vi "test_Error Code Channel Waveform Outgoing.vi"(8 "error in (no error)":errorcluster, 11 "TestCase in":refnum<class "FPGA Addon DMA Waveform Status Channel System Tests.lvclass">) -> (0 "error out":errorcluster, 3 "TestCase out":refnum<class "FPGA Addon DMA Waveform Status Channel System Tests.lvclass">)   [LabVIEW 2018, in "FPGA Addon DMA Waveform Status Channel System Tests.lvclass"]
uses:
  FPGA Addon DMA Waveform Status Channel System Tests.lvclass
  <vilib>/addons/_JKI Toolkits/VI Tester/TestCase.llb/TestCase.lvclass
  C:/Program Files (x86)/National Instruments/LabVIEW 2018/vi.lib/addons/_JKI Toolkits/VI Tester/TestCase.llb/TestCase.lvclass
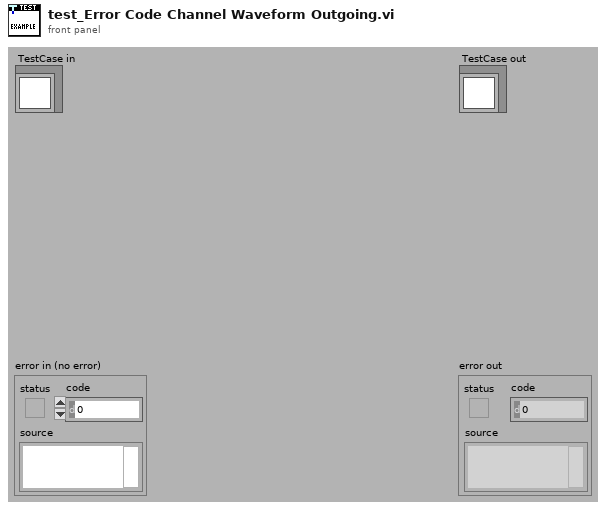
[diagram p1: front panel]
types:
  T1 = typedef "NI_VS Workspace ExecutionAPI.lvlib/WorkspaceAPI.ctl" = refnum<k24>
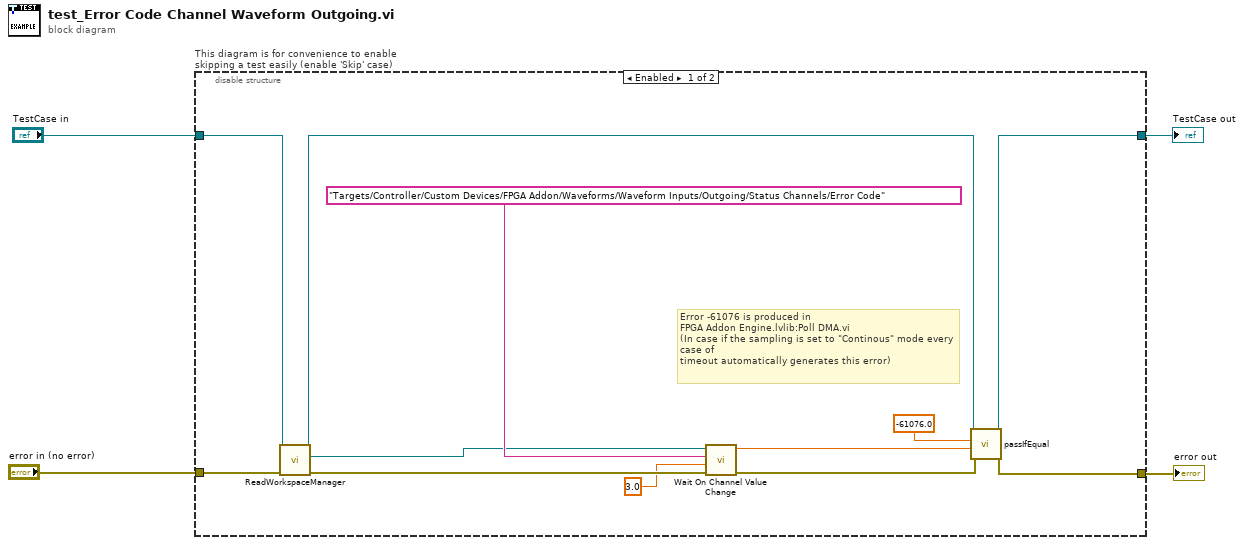
[diagram p0: block diagram]
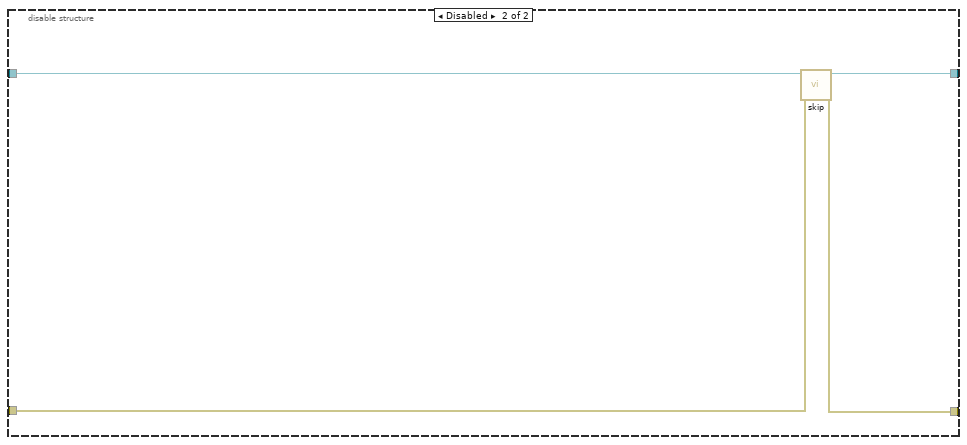
[diagram p2: hidden frame]
diagram:
  n1 = disable-structure "This diagram is for convenience to enable skipping a test easily (enable 'Skip' case)" shown="Enabled" {
    disable-tunnel: "TestCase in" -> [w13 w20]
    disable-tunnel: [w16 w18] -> w1
    disable-tunnel: [w15 w19] -> w3
    disable-tunnel: "error in (no error)" -> [w12 w17]
    frame Enabled {
      # "Error -61076 is produced in \nFPGA Addon Engine.lvlib:Poll DMA.vi\n(In case if the sampling is set to \"Continous\" mode every case of \ntimeout automatically generates this error)"
      n2 = call-dynamic "ReadWorkspaceManager.vi"("error in (no error)"=w12, "VeriStand Test Case in"=w13) -> ("error out"=w10:errorcluster, "Workspace"=w8:T1, "VeriStand Test Case out"=w11:refnum<class "FPGA Addon DMA Waveform Status Channel System Tests.lvclass">)  [unwired: 7 in]
      n3 = call "Wait On Channel Value Change.vi"("error in (no error)"=w10, "Time to Wait"=3.0, "Channel"="Targets/Controller/Custom Devices/FPGA Addon/Waveforms/Waveform Inputs/Outgoing/Status Channels/Error Code", ".NET Refnum in"=w8) -> ("error out"=w7:errorcluster, "Value"=w6:dbl)  [unwired: 6 in]
      n4 = call-dynamic "passIfEqual.vi"("error in (no error)"=w7, "y"=w6, "x"=-61076.0 ("Value"), "TestCase in"=w11) -> ("error out"=w15:errorcluster, "TestCase out"=w16:refnum<class "FPGA Addon DMA Waveform Status Channel System Tests.lvclass">)  [unwired: 6 in]
    }
    frame Disabled {
      # "skip test result while test is under development"
      n5 = call <vilib>:"skip.vi"("error in (no error)"=w17, "TestCase in"=w20) -> ("error out"=w19:errorcluster, "TestCase out"=w18:refnum<class "FPGA Addon DMA Waveform Status Channel System Tests.lvclass">)  [unwired: 8 in]
    }
  }
  "error out" <- w3
  "TestCase out" <- w1
